vi "close.vi"(8 "error in (no error)":errorcluster, 11 "Mockbus in":refnum<class "Mockbus.lvclass">) -> (0 "error out":errorcluster, 3 "Mockbus out":refnum<class "Mockbus.lvclass">)   [LabVIEW 2015, in "RTMockbus.lvlib" / "Mockbus.lvclass"]
uses:
  Mockbus.lvclass
  Mockbus.lvclass/Mockbus.ctl
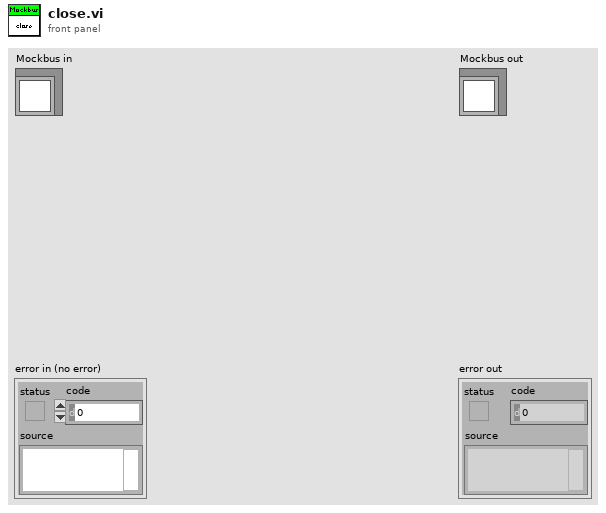
[diagram p1: front panel]
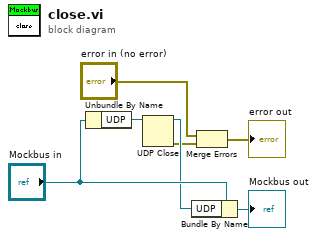
[diagram p0: block diagram]
diagram:
  n1 = Unbundle By Name("Mockbus in") -> ("UDP"=w5:refnum<k16>)
  n2 = UDP Close(connection ID=w5) -> (connection ID out=w4:refnum<k16>, error out=w3:errorcluster)  [unwired: 1 in]
  n3 = Bundle By Name(cluster="Mockbus in", "UDP"=w4) -> (→"Mockbus out":refnum<class "Mockbus.lvclass">)
  n4 = Merge Errors("error in (no error)", w3) -> (→"error out":errorcluster)
